vi "writeFactCorrec.vi"(8 "error in (no error)":errorcluster, 10 "factor_correccion":dbl=1.0) -> (0 "error out":errorcluster, 3 "NEXUS out":refnum<class "NEXUS.lvclass">)   [LabVIEW 2019, in "NEXUS.lvclass"]
uses:
  NEXUS.lvclass
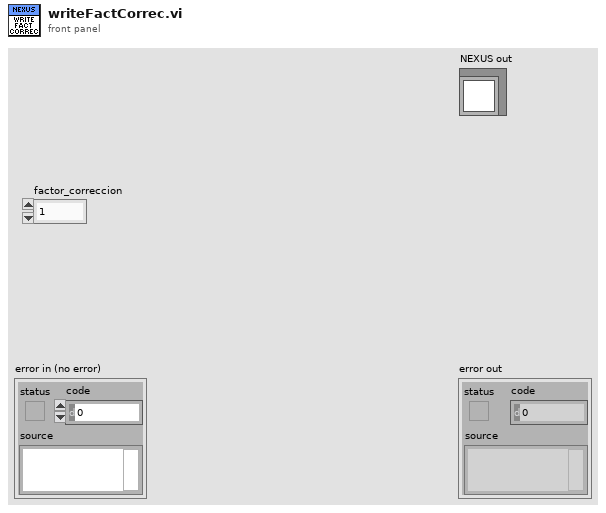
[diagram p1: front panel]
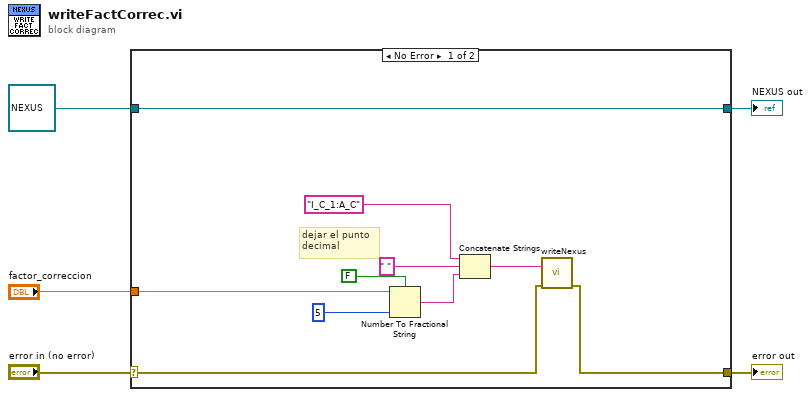
[diagram p0: block diagram]
diagram:
  n1 = case shown="No Error" "error in (no error)" {
    selector: "error in (no error)" -> [w7 w17]
    tunnel: [w6 w17] -> w4
    tunnel: [w15 w16] -> w2
    tunnel: refnum<class "NEXUS.lvclass"> refnum ("NEXUS in") -> [w15 w16]
    tunnel: "factor_correccion" -> [w8 _]
    frame No Error {
      # "dejar el punto \ndecimal"
      n2 = Number To Fractional String(use system decimal point (T)=FALSE, number=w8, precision (6)=i16 5) -> (F-format string=w14:string)  [unwired: 1 in]
      n3 = Concatenate Strings("I_C_1:A_C" ("Command"), " " ("string"), w14) -> (w13:string)
      n4 = call "writeNexus.vi"("error in (no error)"=w7, "Command"=w13) -> ("error out"=w6:errorcluster)  [unwired: 8 in, 1 out]
    }
    frame Error {
    }
  }
  "error out" <- w4
  "NEXUS out" <- w2
